vi "Data View Analysis.vi"() -> ()   [LabVIEW 2020]
panel:
  out "x-scale":dbl=1.0
  out "data cluster":cluster{"all data":dbl[][]}[](array[cluster])
  in  "data beautifier":bool
  out "y-scale factor":dbl format="%#_6e"
  out "Scale 2":u16(ring) items=["no scaling", "universal scale", "1st row", "matrix", "frequency (matrix)", "freq. 1st col. (real 1, im 1, re 2, im 2, ....)"]
  out "selected showfiles":T1(array[cluster]) {"Numeric" format="%#_6f"}
  in  "Analysis":bool
  in  "export data":bool
  in  "X-wave column":u8
  in  "scaling":bool
  out "cue content":T2={"data cluster"=[], "Scale"=0, "scale matrix"=[[1000.0, -1000.0, 200000.0, 1.0, 1.0, 1.0], [2000.0, -500.0, 1000000.0, 0.0, 0.0, 0.0], [5000.0, -1000.0, 1000000.0, 0.0, 0.0, 0.0], [10000.0, -2000.0, 1000000.0, 0.0, 0.0, 0.0], [20000.0, -5000.0, 1000000.0, 0.0, 0.0, 0.0], [500.0, -1000.0, 0.0, 0.0, 0.0, 0.0], [500.0, -40000.0, 0.0, 0.0, 0.0, 0.0], [500.0, -45000.0, 0.0, 0.0, 0.0, 0.0], [500.0, -50000.0, 0.0, 0.0, 0.0, 0.0], [500.0, -1000.0, 0.0, 0.0, 0.0, 0.0], [2000.0, -2000.0, 0.0, 0.0, 0.0, 0.0], [2000.0, -2000.0, 0.0, 0.0, 0.0, 0.0], [4000.0, -4000.0, 0.0, 0.0, 0.0, 0.0], [4000.0, -4000.0, 0.0, 0.0, 0.0, 0.0]], "universal y-scale"=1.0, "data names"=[], "new dataset?"=FALSE, "show files 2"=[]} {"scale matrix" format="%#_6e"; "Scale" items=["no scaling", "1st row", "matrix", "frequency (matrix)", "freq. 1st col. (real 1, im 1, re 2, im 2, ....)"]}
  in  "Y-wave columns":u8[](array[numeric])=[4]
  in  "selection":T3(ring)
  out "XY Graph":T4(graph)
  in  "show files":T5(array[cluster])=[{"String"="20120217.012", "Boolean"=TRUE, "begin"=15, "length"=10000, "y weight"=1.0}]
  in  "import data":bool=TRUE
  in  "stop":bool
  # "show\ntrace?"
  # "scale"
  # "1st elem."
  # "data length"
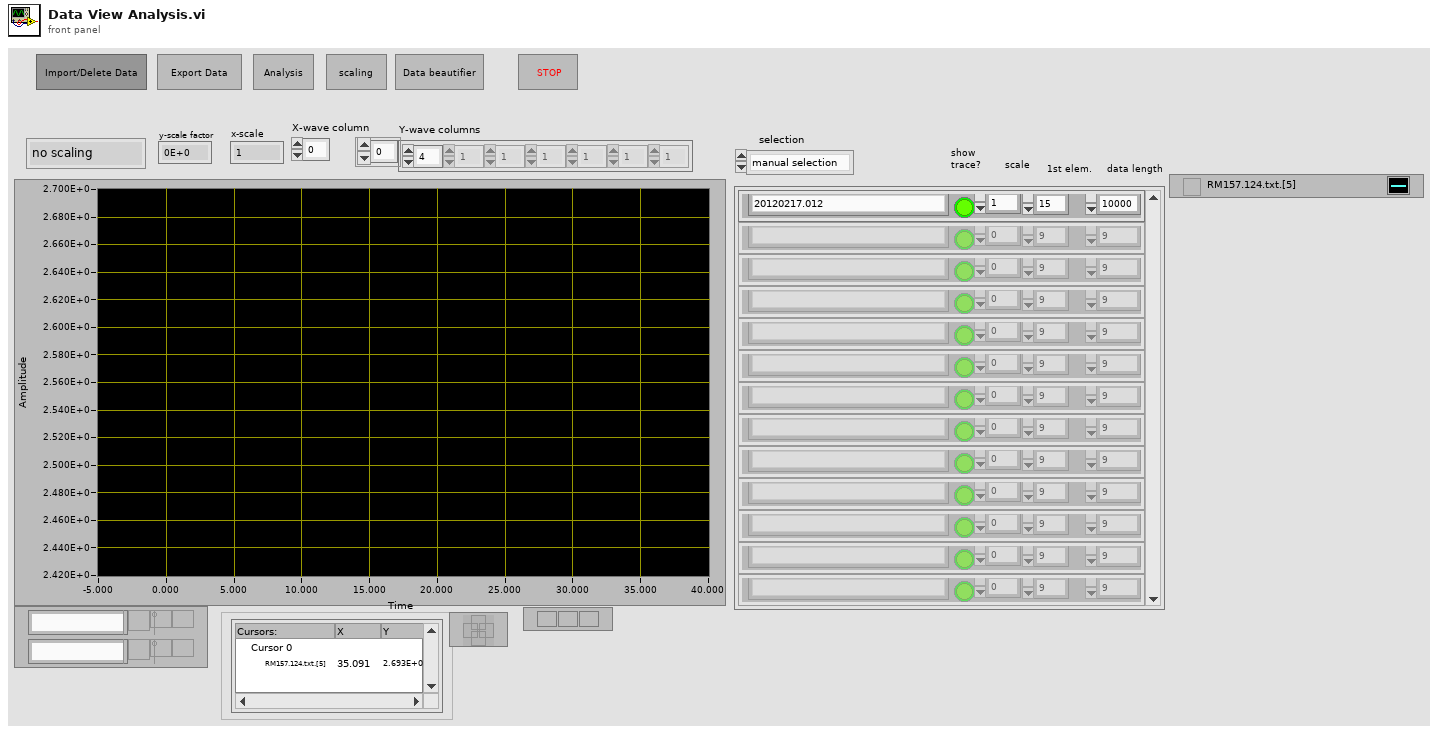
[diagram p1: front panel]
types:
  T1 = cluster{"String":string, "Boolean":bool, "begin":u32, "end":u32, "Numeric":dbl}[]
  T2 = cluster{"data cluster":cluster{"all data":dbl[][]}[], "Scale":u16, "scale matrix":dbl[][], "universal y-scale":dbl, "data names":string[], "new dataset?":bool, "show files 2":cluster{"String":string, "Boolean":bool, "begin":u32, "length":u32, "y weight":dbl}[]}
  T3 = enum16{"manual selection", "select all", "unselect all"}
  T4 = cluster{"indep array (x) out":dbl[], "dep array (y) out":dbl[]}[]
  T5 = cluster{"String":string, "Boolean":bool, "begin":u32, "length":u32, "y weight":dbl}[]
  T6 = cluster{"String":string, "Boolean":bool, "begin":u32, "length":u32, "scale":dbl}[]
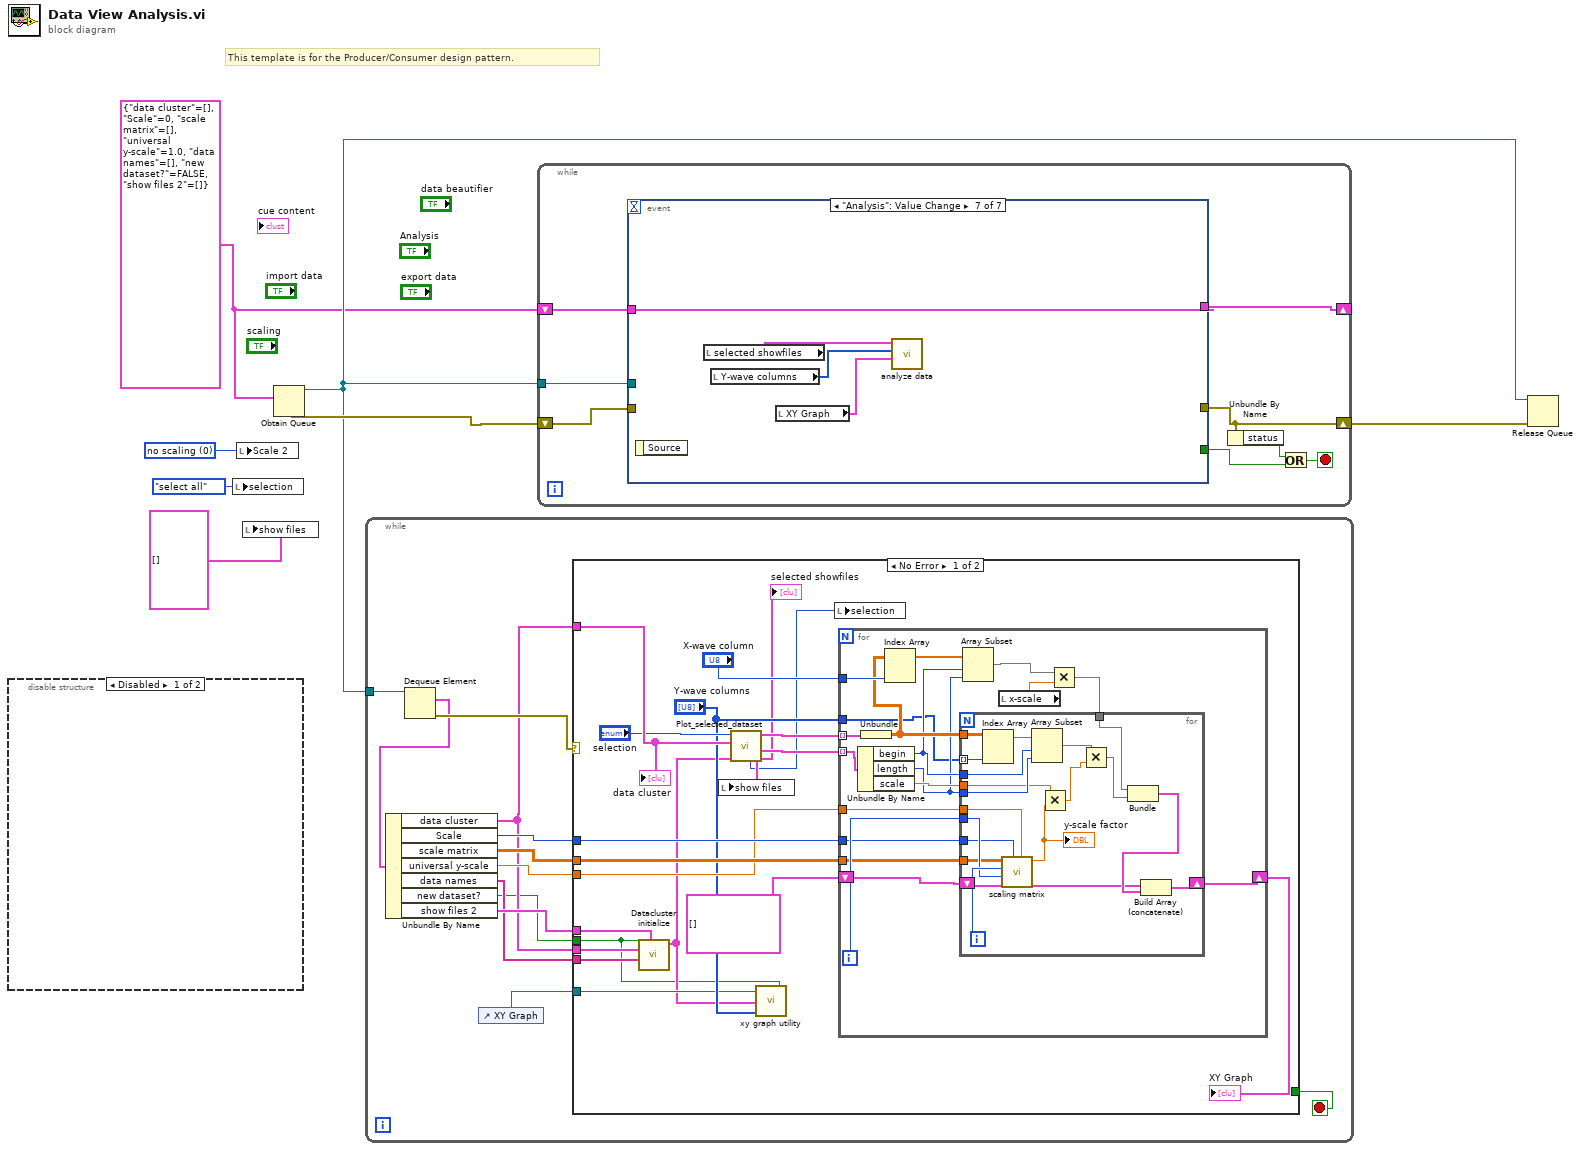
[diagram p0: block diagram]
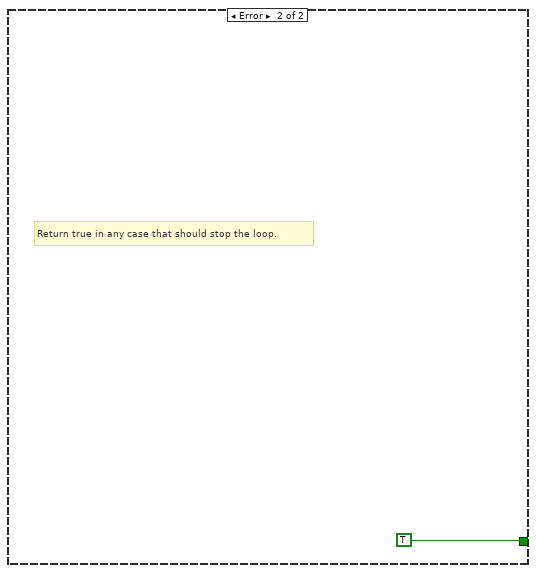
[diagram p3: hidden frame]
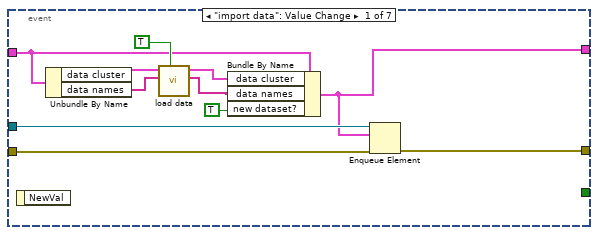
[diagram p4: hidden frame]
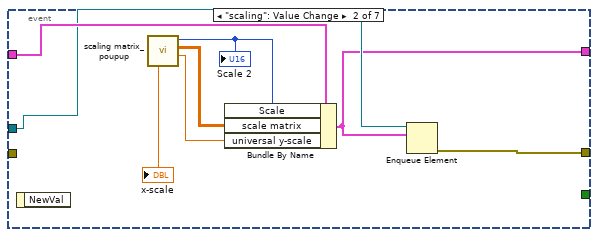
[diagram p5: hidden frame]
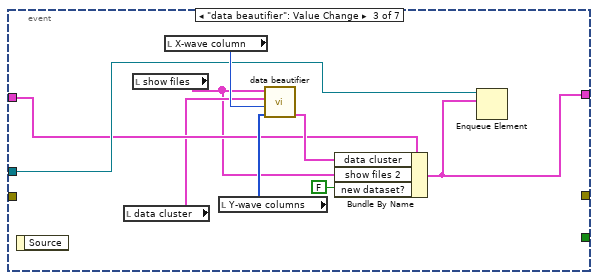
[diagram p6: hidden frame]
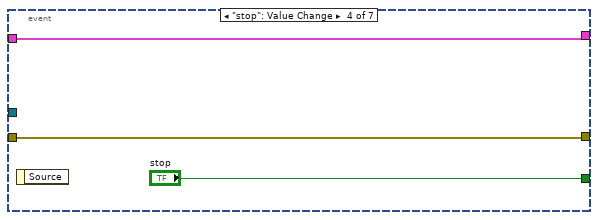
[diagram p7: hidden frame]
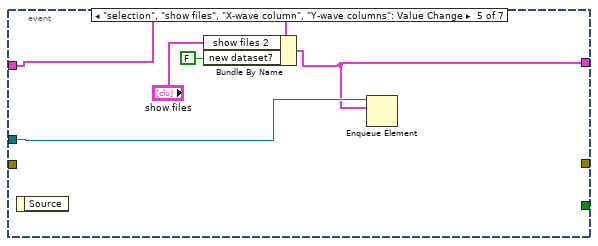
[diagram p8: hidden frame]
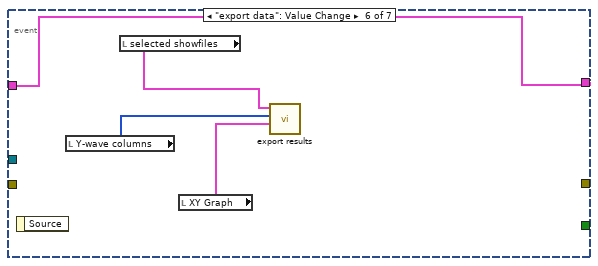
[diagram p9: hidden frame]
diagram:
  w3 = u16 0 items=["no scaling", "1st row", "matrix", "frequency (matrix)", "freq. 1st col. (real 1, im 1, re 2, im 2, ....)"] ("data scaling")
  w4 = T2 {"data cluster"=[], "Scale"=0, "scale matrix"=[], "universal y-scale"=1.0, "data names"=[], "new dataset?"=FALSE, "show files 2"=[]} ("cue content")
  # "This template is for the Producer/Consumer design pattern."
  n1 = disable-structure shown="Disabled" {
    frame Disabled {
    }
    frame Enabled {
    }
  }
  n2 = local write "selection"(T3."select all" ("selection")) -> ()
  n3 = local write "Scale 2"(w3) -> ()
  n4 = local write "show files"(T5 [] ("show files")) -> ()
  n5 = Obtain Queue(element data type=w4) -> (queue out=w5:refnum<queue>, error out=w6:errorcluster)  [unwired: 4 in, 1 out]
  n6 = while {
    tunnel: w5 -> [w19]
    stop <- w17 stop-if-true
    n7 = Dequeue Element(queue=w19) -> (element=w13:T2, error out=w18:errorcluster)  [unwired: 2 in, 2 out]
    n8 = Unbundle By Name(w13) -> ("data cluster"=w10:cluster{"all data":dbl[][]}[], "Scale"=w15:u16, "scale matrix"=w16:dbl[][], "universal y-scale"=w14:dbl, "data names"=w11:string[], "new dataset?"=w9:bool, "show files 2"=w12:T5)
    n9 = control-ref of="XY Graph"() -> (w8:refnum<vi>)
    n10 = case shown="No Error" w18 {
      tunnel: w10 -> [w39 _]
      tunnel: [_ TRUE] -> w17
      tunnel: w16 -> [w38 _]
      tunnel: w15 -> [w37 _]
      tunnel: w14 -> [w36 _]
      tunnel: w12 -> [w30 _]
      tunnel: w11 -> [w29 _]
      tunnel: w10 -> [w28 _]
      tunnel: w9 -> [w20 _]
      tunnel: w8 -> [w26 _]
      frame No Error {
        n11 = call "Datacluster initialize.vi"("show files in"=w30, "data names"=w29, "data cluster"=w28, "reset"=w20) -> ("show files out"=w24:cluster{"String":string, bool, i32, i32, dbl}[])  [unwired: 7 in]
        n12 = call "Plot_selected_dataset.vi"("selection"="selection", "input xy data arrays"=w39, "file names and switch"=w24) -> ("show files out"=w23:T1, "default selection"=w22:T3, "selected xy data arrays"=w34:cluster{"all rows":dbl[][]}[], "selected files2"=w25:T6, "selected showfiles"=→"selected showfiles":T1)  [unwired: 2 out]
        n13 = local write "show files"(w23) -> ()
        n14 = call "xy graph utility.vi"("redraw?"=w20, "y-wave columns"="Y-wave columns", "show files"=w24, "XYGraph Refnum"=w26) -> ()  [unwired: 1 in]
        n15 = local write "selection"(w22) -> ()
        n16 = for {
          tunnel: w34 -> [w56] mode=indexing
          tunnel: w25 -> [w57] mode=indexing
          tunnel: w38 -> [w53]
          tunnel: w37 -> [w52]
          tunnel: w36 -> [w51]
          tunnel: "X-wave column" -> [w50]
          shift-right: [w45] -> w31
          shift-left: T4 [] -> [w44]
          tunnel: "Y-wave columns" -> [w43]
          i -> [w55]
          n17 = Unbundle By Name(w57) -> ("begin"=w47:u32, "length"=w46:u32, "scale"=w54:dbl)
          n18 = Unbundle(w56) -> ("all rows"=w49:dbl[][])
          n19 = Index Array(array=w49, index (col)=w50) -> (element=w48:dbl[])  [unwired: 1 in]
          n20 = Array Subset(array=w48, index=w47, length=w46) -> (w42:dbl[])
          n21 = local read "x-scale"() -> (w40:dbl)
          n22 = Multiply(x=w42, y=w40) -> (x*y=w41:dbl[])
          n23 = for {
            tunnel: w49 -> [w76]
            tunnel: w43 -> [w75] mode=indexing
            tunnel: w47 -> [w73]
            tunnel: w46 -> [w72]
            tunnel: w55 -> [w69]
            tunnel: w54 -> [w68]
            tunnel: w53 -> [w66]
            tunnel: w52 -> [w65]
            tunnel: w51 -> [w64]
            tunnel: w41 -> [w60]
            shift-right: [w61] -> w45
            shift-left: w44 -> [w62]
            i -> [w70]
            n24 = Index Array(array=w76, index (col)=w75) -> (element=w74:dbl[])  [unwired: 1 in]
            n25 = call "scaling matrix.vi"("universal y-scale"=w64, "Scale"=w65, "row index"=w69, "col index"=w70, "scale matrix"=w66) -> ("scale\nfactor"=w58:dbl)  [unwired: 6 in]
            "y-scale factor" <- w58
            n26 = Array Subset(array=w74, index=w73, length=w72) -> (w71:dbl[])
            n27 = Multiply(x=w68, y=w58) -> (x*y=w67:dbl)
            n28 = Multiply(x=w71, y=w67) -> (x*y=w59:dbl[])
            n29 = Bundle(w60, w59) -> (w63:cluster{dbl[], dbl[]})  [unwired: 1 out]
            n30 = Build Array (concatenate)(w62, w63) -> (w61:T4)
          }
        }
        "XY Graph" <- w31
        "data cluster" <- w39
      }
      frame Error {
        # "Return true in any case that should stop the loop."
      }
    }
  }
  n31 = while {
    shift-right: [w83] -> w7
    shift-left: w6 -> [w80]
    tunnel: w5 -> [w79]
    shift-right: [w78] -> _
    shift-left: w4 -> [w81]
    stop <- w84 stop-if-true
    n32 = event shown="[6] \"Analysis\": Value Change" {
      selector: _ -> [_ _ _ _ _ _ _]
      dyn-events: _ -> [_ _ _ _ _ _ _]
      timeout: _ -> [_ _ _ _ _ _ _]
      tunnel: w80 -> [w96 _ _ w115 _ _ _]
      tunnel: [w95 w104 _ w115 _ _ _] -> w83
      tunnel: [_ _ _ "stop" _ _ _] -> w85
      tunnel: w81 -> [w88 w101 w108 w114 w120 w122 w129]
      tunnel: w79 -> [w93 w100 w109 _ w121 _ _]
      tunnel: [w92 w99 w112 w114 w119 w122 w129] -> w78
      event "import data": Value Change {
        n33 = event-data() -> ()  [unwired: 1 in, 1 out]
        n34 = Unbundle By Name(w88) -> ("data cluster"=w87:cluster{"all data":dbl[][]}[], "data names"=w86:string[])
        n35 = call "load data.vi"("Append dataset"=TRUE, "existing file numbers"=w86, "existing data cluster"=w87) -> ("data names"=w91:string[], "data cluster"=w94:cluster{"all data":dbl[][]}[])  [unwired: 7 in]
        n36 = Bundle By Name(cluster=w88, "data cluster"=w94, "data names"=w91, "new dataset?"=TRUE) -> (w92:T2)
        n37 = Enqueue Element(queue=w93, element=w92, error in (no error)=w96) -> (error out=w95:errorcluster)  [unwired: 1 in, 2 out]
      }
      event "scaling": Value Change {
        n38 = event-data() -> ()  [unwired: 1 in, 1 out]
        n39 = call "scaling matrix_poupup.vi"() -> ("scale\nfactor"=w98:dbl, "scale matrix 2"=w102:dbl[][], "Scale 2"=w103:u16, "x-scale"=→"x-scale":dbl)  [unwired: 4 in, 1 out]
        "Scale 2" <- w103
        n40 = Bundle By Name(cluster=w101, "Scale"=w103, "scale matrix"=w102, "universal y-scale"=w98) -> (w99:T2)
        n41 = Enqueue Element(queue=w100, element=w99) -> (error out=w104:errorcluster)  [unwired: 2 in, 2 out]
      }
      event "data beautifier": Value Change {
        n42 = event-data() -> ()  [unwired: 1 in, 1 out]
        n43 = local read "data cluster"() -> (w107:cluster{"all data":dbl[][]}[])
        n44 = local read "show files"() -> (w106:T5)
        n45 = local read "X-wave column"() -> (w110:u8)
        n46 = local read "Y-wave columns"() -> (w111:u8[])
        n47 = call "data beautifier.vi"("Y-wave columns"=w111, "X-wave column"=w110, "data cluster"=w107, "show files"=w106) -> ("result data cluster"=w113:cluster{"all rows":dbl[][]}[])  [unwired: 5 in]
        n48 = Bundle By Name(cluster=w108, "data cluster"=w113, "show files 2"=w106, "new dataset?"=FALSE) -> (w112:T2)
        n49 = Enqueue Element(queue=w109, element=w112) -> ()  [unwired: 2 in, 3 out]
      }
      event "stop": Value Change {
        n50 = event-data() -> ()  [unwired: 1 in, 1 out]
      }
      event "selection", "show files", "X-wave column", "Y-wave columns": Value Change {
        n51 = event-data() -> ()  [unwired: 1 in, 1 out]
        n52 = Bundle By Name(cluster=w120, "show files 2"="show files", "new dataset?"=FALSE) -> (w119:T2)
        n53 = Enqueue Element(queue=w121, element=w119) -> ()  [unwired: 2 in, 3 out]
      }
      event "export data": Value Change {
        n54 = event-data() -> ()  [unwired: 1 in, 1 out]
        n55 = local read "Y-wave columns"() -> (w124:u8[])
        n56 = local read "selected showfiles"() -> (w123:T1)
        n57 = local read "XY Graph"() -> (w125:T4)
        n58 = call "export results.vi"("Graph array"=w125, "Y-columns"=w124, "selected files2"=w123) -> ()  [unwired: 9 in]
      }
      event "Analysis": Value Change {
        n59 = event-data() -> ()  [unwired: 1 in, 1 out]
        n60 = local read "selected showfiles"() -> (w128:T1)
        n61 = local read "Y-wave columns"() -> (w127:u8[])
        n62 = local read "XY Graph"() -> (w126:T4)
        n63 = call "analyze data.vi"("Graph array"=w126, "Y-columns"=w127, "selected files2"=w128) -> ()  [unwired: 9 in]
      }
    }
    n64 = Unbundle By Name(w83) -> ("status"=w82:bool)
    n65 = Or(x=w82, y=w85) -> (x .or. y?=w84:bool)
  }
  n66 = Release Queue(queue=w5, error in (no error)=w7) -> ()  [unwired: 1 in, 3 out]
